vi "Video record flag initialise.vi"(8 "error in (no error)":errorcluster) -> (0 "error out (no error)":errorcluster)   [LabVIEW 2013]
uses:
  typedefs/Functions enum.ctl
  Global Variables/General Globals.vi
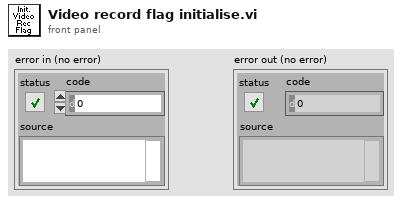
[diagram p1: front panel]
types:
  T1 = typedef "Functions enum.ctl" = enum16{"Create", "Start", "Write", "Stop", "Clear"}
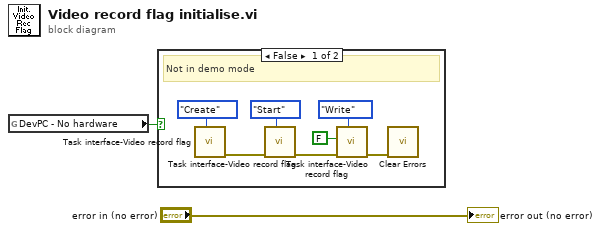
[diagram p0: block diagram]
diagram:
  n1 = global read "General Globals.vi" "DevPC - No hardware"() -> (w1:bool)
  n2 = case shown="False" w1 {
    frame False {
      # "Not in demo mode"
      n3 = call "Task interface-Video record flag.vi"("Function"=Functions_enum."Create") -> ("error out"=w6:errorcluster)  [unwired: 10 in]
      n4 = call "Task interface-Video record flag.vi"("Function"=Functions_enum."Start", "error in"=w6) -> ("error out"=w8:errorcluster)  [unwired: 9 in]
      n5 = call "Task interface-Video record flag.vi"("Function"=Functions_enum."Write", "error in"=w8, "DO value"=FALSE) -> ("error out"=w3:errorcluster)  [unwired: 8 in]
      n6 = call <vilib>:"Clear Errors.vi"("error in (no error)"=w3) -> ()  [unwired: 6 in, 1 out]
    }
    frame True {
      # "Demo mode"
    }
  }
  "error out (no error)" <- "error in (no error)"
